vi "Begin.vi"() -> (0 "error out":errorcluster)   [LabVIEW 2019]
doc: "Called before other user functions, this VI is expected to open initial I/O refnums, load in file data, and do all program initialization. Notice that the <B>error out</B> terminal is simply used for data flow. Wiring it to other structures or subVIs ensures that this VI runs first."
uses:
  <vilib>/Rock Robotics/WPI/DriverStation/WPI_DriverStationRobotMode2.ctl
  <vilib>/Rock Robotics/WPI/Joystick/WPI_JoystickDeviceEnum.ctl
  <vilib>/Rock Robotics/WPI/ThirdParty/Phoenix-LabVIEW/Motor Controller/Controls/CTRE_Phoenix_MotorControl_MotionProfileTrajectoryPoint.ctl
  Robot Global Data.vi
  <vilib>/Rock Robotics/WPI/ThirdParty/Phoenix-LabVIEW/Pigeon IMU/CTRE_PigeonIMU_Open_TalonSRX.vi
  <vilib>/Utility/file.llb/Read Delimited Spreadsheet (DBL).vi
  <vilib>/Rock Robotics/WPI/ThirdParty/Phoenix-LabVIEW/Motor Controller/Closed Loop/Motion Profile/CTRE_Phoenix_MotorControl_BufferedTrajectoryPointStream_WriteAll.vi
panel:
  in  "error in":errorcluster
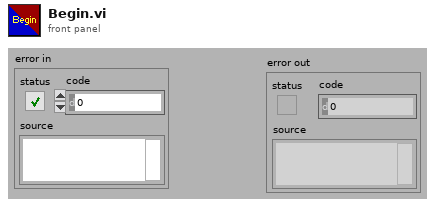
[diagram p1: front panel]
types:
  T1 = typedef "WPI_JoystickDeviceEnum.ctl" = enum16{"USB 0", "USB 1", "USB 2", "USB 3", "USB 4", "USB 5"}
  T2 = typedef "WPI_DriverStationRobotMode2.ctl" = enum16{"Autonomous Disabled", "Autonomous Enabled", "Teleop Disabled", "Teleop Enabled", "Disconnected", "Finish", "Test Disabled", "Test Enabled", "Emergency Stopped"}
  T3 = typedef "WPI_JoystickDevRef.ctl" = cluster{"Device":T1}
  T4 = typedef "WPI_MotorControlDeviceRef.ctl" = cluster{"DeviceStatus":errorcluster, "Type":T5, "PWM":cluster{"PWM Channel":T6, "DeadBand":T7}, "CAN":cluster{"Device Number":u8, "SetOutput VI Ref":variant, "GetOutput VI Ref":variant, "Enable VI Ref":variant, "Disable VI Ref":variant, "Data":variant}, "Invert":bool, "DIO PWM":cluster{"PWM \"Enable\" Channel":T6, "DIOChannel":T8, "PWM Rate":dbl}}
  T5 = typedef "WPI_MotorControlType.ctl" = enum16{"PWM", "CAN", "DIO PWM"}
  T6 = typedef "FPGA_DIOPWMChannel.ctl" = enum8{"PWM 0", "PWM 1", "PWM 2", "PWM 3", "PWM 4", "PWM 5", "PWM 6", "PWM 7", "PWM 8", "PWM 9", "PWM MXP 0", "PWM MXP 1", "PWM MXP 2", "PWM MXP 3", "PWM MXP 4", "PWM MXP 5", "PWM MXP 6", "PWM MXP 7", "PWM MXP 8", "PWM MXP 9", "Invalid"}
  T7 = typedef "WPI_PWMDeadband.ctl" = cluster{"Name":string, "maxPositivePwm":i32, "minPositivePwm":i32, "centerPwm":i32, "maxNegativePwm":i32, "minNegativePwm":i32, "angularRange":u16}
  T8 = typedef "FPGA_DIOChannel.ctl" = enum8{"DIO 0", "DIO 1", "DIO 2", "DIO 3", "DIO 4", "DIO 5", "DIO 6", "DIO 7", "DIO 8", "DIO 9", "DIO MXP 0", "DIO MXP 1", "DIO MXP 2", "DIO MXP 3", "DIO MXP 4", "DIO MXP 5", "DIO MXP 6", "DIO MXP 7", "DIO MXP 8", "DIO MXP 9", "DIO MXP 10", "DIO MXP 11", "DIO MXP 12", "DIO MXP 13", "DIO MXP 14", "DIO MXP 15", "SPI Port CS1", "SPI Port CS2", "SPI Port CS3", "SPI Port MISO", "SPI Port MOSI", "Invalid"}
  T9 = typedef "CTRE_Phoenix_MotorControl_MotionProfileTrajectoryPoint.ctl" = cluster{"Position":dbl, "Velocity":dbl, "Arbitrary Feed Forward":dbl, "Auxiliary Position":dbl, "Auxiliary Velocity":dbl, "Auxiliary Arbitrary Feed Forward":dbl, "Profile Slot Select":i32, "Auxiliary Profile Slot Select":i32, "isLastPoint?":bool, "Zero Position?":bool, "durationMs":u32, "Use Aux PID?":bool}
  T10 = typedef "CTRE_PigeonIMU_DeviceRef.ctl" = cluster{"DeviceStatus":errorcluster, "Device Number":u8, "Type":T11, "Device ID":u32, "Handle":u64, "UsageFrame":u32, "Library Path":path}
  T11 = typedef "CTRE_PigeonIMU_ConnectionType.ctl" = u32
  T12 = typedef "CTRE_Phoenix_MotorControl_BufferedTrajectoryPointStream_DeviceRef.ctl" = cluster{"Handle":u64, "Library Path":path}
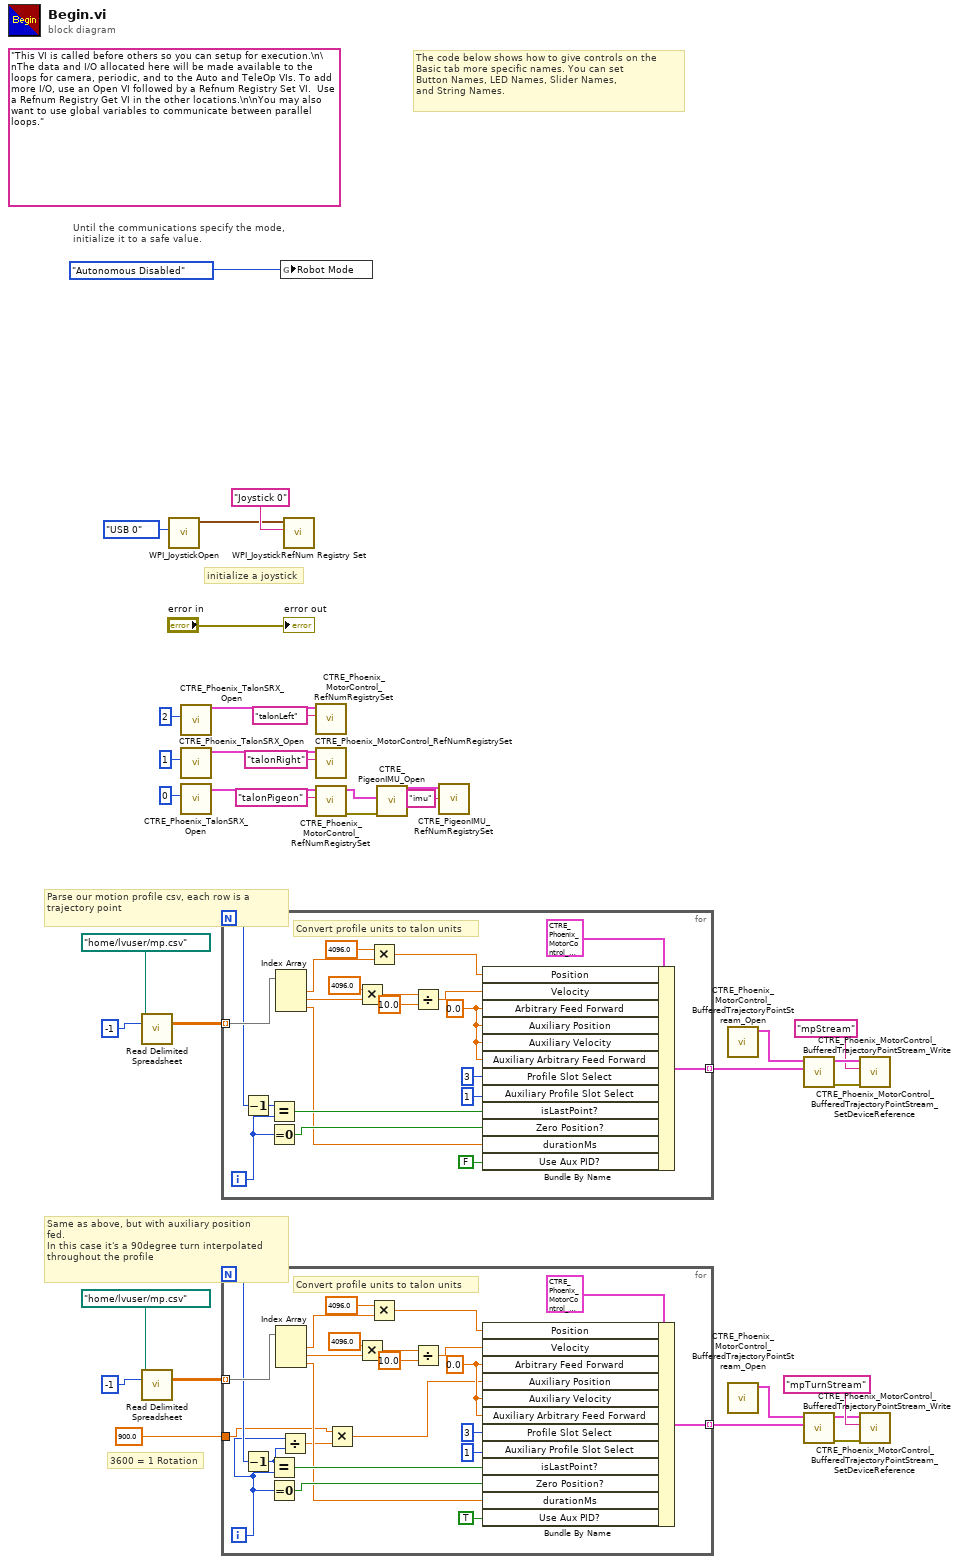
[diagram p0: block diagram]
diagram:
  (unwired) "This VI is called before others so you can setup for execution.\n\nThe data and I/O allocated here will be made available to the loops for camera, periodic, and to the Auto and TeleOp VIs. To add more I/O, use an Open VI followed by a Refnum Registry Set VI.  Use a Refnum Registry Get VI in the other locations.\n\nYou may also want to use global variables to communicate between parallel loops."
  # "3600 = 1 Rotation"
  # "Same as above, but with auxiliary position\nfed.\nIn this case it's a 90degree turn interpolated throughout the profile"
  # "Parse our motion profile csv, each row is a trajectory point"
  # "The code below shows how to give controls on the\nBasic tab more specific names. You can set\nButton Names, LED Names, Slider Names,\nand String Names."
  # "initialize a joystick"
  # "Until the communications specify the mode,\ninitialize it to a safe value."
  n1 = call-poly <vilib>:"Read Delimited Spreadsheet.vi"("file path (dialog if empty)"=path "/home/lvuser/mp.csv" ("file path (use dialog)"), "number of rows (all:-1)"=-1) -> ("all rows"=w17:dbl[][])  [unwired: 8 in, 5 out]
  n2 = call-poly <vilib>:"Read Delimited Spreadsheet.vi"("file path (dialog if empty)"=path "/home/lvuser/mp.csv" ("file path (use dialog)"), "number of rows (all:-1)"=-1) -> ("all rows"=w6:dbl[][])  [unwired: 8 in, 5 out]
  n3 = call <vilib>:"WPI_JoystickOpen.vi"("JoystickDevice"=WPI_JoystickDeviceEnum."USB 0") -> ("JoystickDevRef"=w34:T3)  [unwired: 10 in]
  n4 = call <vilib>:"CTRE_Phoenix_TalonSRX_Open.vi"("Device Number"=u8 2) -> ("CAN Talon SRX Ref"=w29:T4)  [unwired: 9 in, 1 out]
  n5 = call <vilib>:"CTRE_Phoenix_TalonSRX_Open.vi"("Device Number"=u8 1) -> ("CAN Talon SRX Ref"=w28:T4)  [unwired: 9 in, 1 out]
  n6 = call <vilib>:"CTRE_Phoenix_TalonSRX_Open.vi"("Device Number"=u8 0) -> ("CAN Talon SRX Ref"=w27:T4)  [unwired: 9 in, 1 out]
  n7 = for {
    N -> [w49]
    tunnel: w17 -> [w55] mode=indexing
    tunnel: [w45] -> w16 mode=indexing
    i -> [w48]
    w54 = 0.0 ("Arbitrary Feed Forward")
    # "Convert profile units to talon units"
    n8 = Decrement(x=w49) -> (x-1=w50:i32)
    n9 = Equal?(x=w50, y=w48) -> (x = y?=w51:bool)
    n10 = Equal To 0?(x=w48) -> (x = 0?=w47:bool)
    n11 = Index Array(array=w55) -> (element #1=w43:dbl, element #2=w37:dbl, element #3=w44:dbl)  [unwired: 3 in]
    n12 = Multiply(x=4096.0, y=w37) -> (x*y=w39:dbl)
    n13 = Multiply(x=4096.0, y=w43) -> (x*y=w41:dbl)
    n14 = Divide(x=w39, y=10.0) -> (x/y=w36:dbl)
    n15 = Bundle By Name(cluster=T9 {"Position"=0.0, "Velocity"=0.0, "Arbitrary Feed Forward"=0.0, "Auxiliary Position"=0.0, "Auxiliary Velocity"=0.0, "Auxiliary Arbitrary Feed Forward"=0.0, "Profile Slot Select"=0, "Auxiliary Profile Slot Select"=0, "isLastPoint?"=FALSE, "Zero Position?"=FALSE, "durationMs"=0, "Use Aux PID?"=FALSE} ("Trajectory Point"), "Position"=w41, "Velocity"=w36, "Arbitrary Feed Forward"=w54, "Auxiliary Position"=w54, "Auxiliary Velocity"=w54, "Auxiliary Arbitrary Feed Forward"=w54, "Profile Slot Select"=3, "Auxiliary Profile Slot Select"=1, "isLastPoint?"=w51, "Zero Position?"=w47, "durationMs"=w44, "Use Aux PID?"=FALSE) -> (w45:T9)
  }
  n16 = for {
    N -> [w74]
    tunnel: w6 -> [w79] mode=indexing
    tunnel: [w71] -> w7 mode=indexing
    tunnel: 900.0 ("x") -> [w58]
    i -> [w61]
    w78 = 0.0 ("Arbitrary Feed Forward")
    # "Convert profile units to talon units"
    n17 = Decrement(x=w74) -> (x-1=w60:i32)
    n18 = Equal?(x=w60, y=w61) -> (x = y?=w75:bool)
    n19 = Equal To 0?(x=w61) -> (x = 0?=w73:bool)
    n20 = Index Array(array=w79) -> (element #1=w69:dbl, element #2=w63:dbl, element #3=w70:dbl)  [unwired: 3 in]
    n21 = Divide(x=w61, y=w60) -> (x/y=w59:dbl)
    n22 = Multiply(x=w58, y=w59) -> (x*y=w57:dbl)
    n23 = Multiply(x=4096.0, y=w63) -> (x*y=w65:dbl)
    n24 = Multiply(x=4096.0, y=w69) -> (x*y=w67:dbl)
    n25 = Divide(x=w65, y=10.0) -> (x/y=w62:dbl)
    n26 = Bundle By Name(cluster=T9 {"Position"=0.0, "Velocity"=0.0, "Arbitrary Feed Forward"=0.0, "Auxiliary Position"=0.0, "Auxiliary Velocity"=0.0, "Auxiliary Arbitrary Feed Forward"=0.0, "Profile Slot Select"=0, "Auxiliary Profile Slot Select"=0, "isLastPoint?"=FALSE, "Zero Position?"=FALSE, "durationMs"=0, "Use Aux PID?"=FALSE} ("Trajectory Point"), "Position"=w67, "Velocity"=w62, "Arbitrary Feed Forward"=w78, "Auxiliary Position"=w57, "Auxiliary Velocity"=w78, "Auxiliary Arbitrary Feed Forward"=w78, "Profile Slot Select"=3, "Auxiliary Profile Slot Select"=1, "isLastPoint?"=w75, "Zero Position?"=w73, "durationMs"=w70, "Use Aux PID?"=TRUE) -> (w71:T9)
  }
  n27 = global write "Robot Global Data.vi" "Robot Mode"(WPI_DriverStationRobotMode2."Autonomous Disabled" ("Robot Mode")) -> ()
  n28 = call <vilib>:"WPI_JoystickRefNum Registry Set.vi"("refnum name"="Joystick 0", "JoystickDevRef"=w34) -> ()  [unwired: 8 in, 2 out]
  n29 = call <vilib>:"CTRE_Phoenix_MotorControl_RefNumRegistrySet.vi"("refnum name"="talonLeft", "PhoenixMotorControlDevRef"=w29) -> ()  [unwired: 8 in, 2 out]
  n30 = call <vilib>:"CTRE_Phoenix_MotorControl_RefNumRegistrySet.vi"("refnum name"="talonRight", "PhoenixMotorControlDevRef"=w28) -> ()  [unwired: 8 in, 2 out]
  n31 = call <vilib>:"CTRE_Phoenix_MotorControl_RefNumRegistrySet.vi"("refnum name"="talonPigeon", "PhoenixMotorControlDevRef"=w27) -> ("error out"=w23:errorcluster, "PhoenixMotorControlDevRef"=w22:T4)  [unwired: 8 in]
  n32 = call-poly <vilib>:"CTRE_PigeonIMU_Open.vi"("error in"=w23, "CAN Talon SRX Ref"=w22) -> ("PigeonIMUDevRef"=w21:T10)  [unwired: 8 in, 1 out]
  n33 = call <vilib>:"CTRE_PigeonIMU_RefNumRegistrySet.vi"("refnum name"="imu", "PigeonIMUDevRef"=w21) -> ()  [unwired: 8 in, 2 out]
  n34 = call <vilib>:"CTRE_Phoenix_MotorControl_BufferedTrajectoryPointStream_Open.vi"() -> ("BufferedTrajectoryPointStream_DevRef"=w15:T12)  [unwired: 10 in, 1 out]
  n35 = call <vilib>:"CTRE_Phoenix_MotorControl_BufferedTrajectoryPointStream_Open.vi"() -> ("BufferedTrajectoryPointStream_DevRef"=w8:T12)  [unwired: 10 in, 1 out]
  n36 = call-poly <vilib>:"CTRE_Phoenix_MotorControl_BufferedTrajectoryPointStream_Write.vi"("Motion Profile Trajectory Point Array"=w16, "BufferedTrajectoryPointStream_DevRef"=w15) -> ("error out"=w13:errorcluster, "BufferedTrajectoryPointStream_DevRef"=w14:T12)  [unwired: 8 in]
  n37 = call-poly <vilib>:"CTRE_Phoenix_MotorControl_BufferedTrajectoryPointStream_Write.vi"("Motion Profile Trajectory Point Array"=w7, "BufferedTrajectoryPointStream_DevRef"=w8) -> ("error out"=w10:errorcluster, "BufferedTrajectoryPointStream_DevRef"=w9:T12)  [unwired: 8 in]
  n38 = call <vilib>:"CTRE_Phoenix_MotorControl_BufferedTrajectoryPointStream_SetDeviceReference.vi"("error in (no error)"=w13, "refnum name"="mpStream", "BufferedTrajectoryPointStream_DevRef"=w14) -> ()  [unwired: 7 in, 2 out]
  n39 = call <vilib>:"CTRE_Phoenix_MotorControl_BufferedTrajectoryPointStream_SetDeviceReference.vi"("error in (no error)"=w10, "refnum name"="mpTurnStream", "BufferedTrajectoryPointStream_DevRef"=w9) -> ()  [unwired: 7 in, 2 out]
  "error out" <- "error in"
